vi "Test Suite Result Published.vi"(8 "error in (no error)":errorcluster, 11 "Result Observation Test In":refnum<class "Result Observation Test.lvclass">) -> (0 "error out":errorcluster, 3 "Result Observation Test Out":refnum<class "Result Observation Test.lvclass">)   [LabVIEW 2020, in "Result Observation Test.lvclass"]
uses:
  Result Observation Test.lvclass
  C:/Program Files (x86)/National Instruments/LabVIEW 2020/vi.lib/Astemes/LUnit/Test Case.lvclass
  Result/Type.ctl
  LUnit Test Case Tests/LUnit Test Case V2 Test Double/LUnit Test Case V2 Test Double.lvclass
  C:/Git/astemes-lunit/source/Rewrite Project/LUnit Test Case/LUnit Test Case V2.lvclass
  LUnit Test Suite/LUnit Test Suite V2.lvclass
  C:/Git/astemes-lunit/source/Rewrite Project/Run/Runnable.lvclass
  <vilib>/Astemes/LUnit/Test Case.lvclass/Test Case.ctl
  <vilib>/Astemes/LUnit/Set Assertion Type.vi
  <vilib>/Astemes/LUnit/Palette/Pass.vi
  <vilib>/Astemes/LUnit/Palette/Fail.vi
  <vilib>/Astemes/LUnit/Add test result.vi
  <vilib>/Astemes/LUnit/LUnit Record Assertion Result.vi
  <vilib>/Astemes/LUnit/LUnit Aggregate Assertion Results.vi
  <vilib>/Astemes/LUnit/Method Result/LUnit Merge Status.vi
  <vilib>/Astemes/LUnit/LUnit Concatenate result strings.vi
  Mock Result Observer/Mock Result Observer.lvclass
  C:/Git/astemes-lunit/source/Rewrite Project/Result Observer/Result Observer.lvclass
  Result Observation Test.lvclass/Result Observation Test.ctl
  Result/Result.lvlib
  <vilib>/Astemes/LUnit/Test Case.lvclass
  C:/Git/astemes-lunit/source/Rewrite Project/LUnit Test Case Tests/LUnit Test Case V2 Test Double/LUnit Test Case V2 Test Double.lvclass
  C:/Git/astemes-lunit/source/Rewrite Project/Mock Result Observer/Mock Result Observer.lvclass
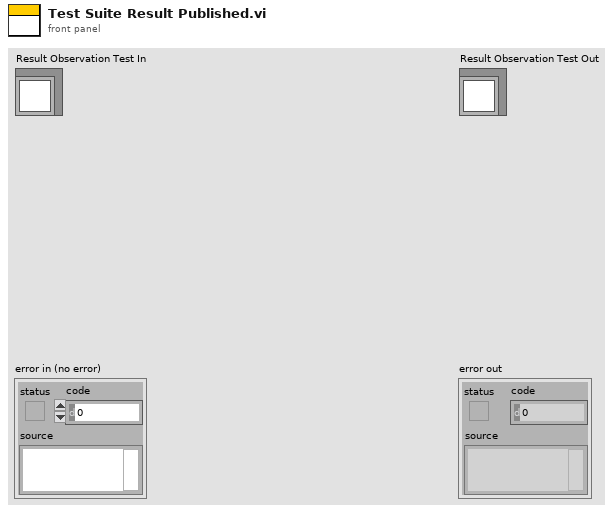
[diagram p1: front panel]
types:
  T1 = typedef "Result.lvlib/Type.ctl" = enum16{"Method", "Case", "Suite", "Pass", "Fail", "Skip", "Pass if", "Fail if", "Pass if Error", "Fail if Error", "Pass if Equal", "Fail if Equal"}
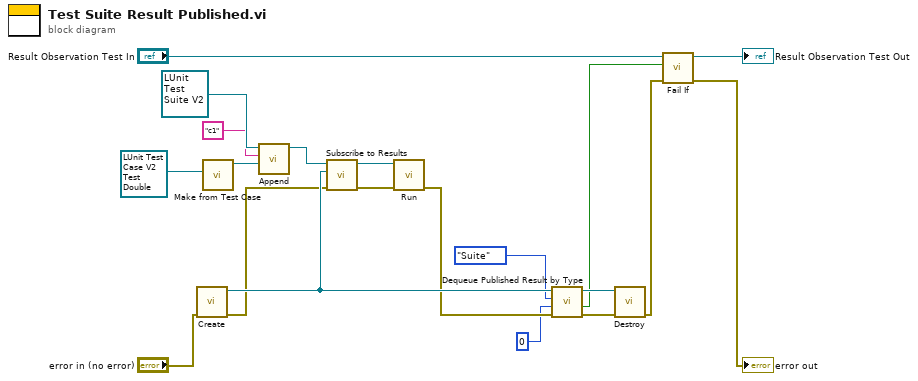
[diagram p0: block diagram]
diagram:
  n1 = call "Create.vi"("error in (no error)"="error in (no error)") -> ("error out"=w5:errorcluster, "Mock Result Observer out"=w16:refnum<class "Mock Result Observer.lvclass">)  [unwired: 9 in]
  n2 = call "Make from Test Case.vi"("LUnit Test Case"=refnum<class "LUnit Test Case V2 Test Double.lvclass"> refnum ("LUnit Test Case V2 Test Double.lvclass")) -> ("LUnit Test Suite V2 out"=w3:refnum<class "LUnit Test Suite V2.lvclass">)  [unwired: 9 in, 1 out]
  n3 = call "Append.vi"("Runnable"=w3, "Name"="c1", "LUnit Test Suite V2 in"=refnum<class "LUnit Test Suite V2.lvclass"> refnum) -> ("LUnit Test Suite V2 out"=w2:refnum<class "LUnit Test Suite V2.lvclass">)  [unwired: 7 in, 1 out]
  n4 = call-dynamic "Subscribe to Results.vi"("error in (no error)"=w5, "Result Observer"=w16, "LUnit Test Suite V2 In"=w2) -> ("error out"=w13:errorcluster, "LUnit Test Suite V2 Out"=w15:refnum<class "LUnit Test Suite V2.lvclass">)  [unwired: 7 in]
  n5 = call-dynamic "Run.vi"("error in (no error)"=w13, "Run in"=w15) -> ("error out"=w12:errorcluster)  [unwired: 8 in, 1 out]
  n6 = call "Dequeue Published Result by Type.vi"("error in (no error)"=w12, "timeout in ms"=0 ("timeout in ms (-1)"), "Result Type"=Type."Suite", "Mock Result Observer In"=w16) -> ("error out"=w18:errorcluster, "timed out?"=w9:bool, "Mock Result Observer Out"=w19:refnum<class "Mock Result Observer.lvclass">)  [unwired: 4 in, 1 out]
  n7 = call "Destroy.vi"("error in (no error)"=w18, "Mock Result Observer in"=w19) -> ("error out"=w8:errorcluster)  [unwired: 9 in]
  n8 = call <vilib>:"Fail If.vi"("error in (no error)"=w8, "Fail?"=w9, "LUnit Test Case In"="Result Observation Test In") -> ("error out"=→"error out":errorcluster, "LUnit Test Case Out"=→"Result Observation Test Out":refnum<class "Result Observation Test.lvclass">)  [unwired: 7 in]
